vi "Post-Init.vi"(8 "error in (no error)":errorcluster, 11 "Pulse Driver in":refnum<class "Pulse Driver.lvclass">) -> (0 "error out":errorcluster, 2 "Init Result":refnum<class "Acquired Result.lvclass">, 3 "Pulse Driver out":refnum<class "Pulse Driver.lvclass">)   [LabVIEW 2019, in "Pulse Driver.lvclass"]
uses:
  Pulse Driver.lvclass
  Instrument Driver/Instrument Driver.lvclass
  Results/Acquired Result/Acquired Result.lvclass
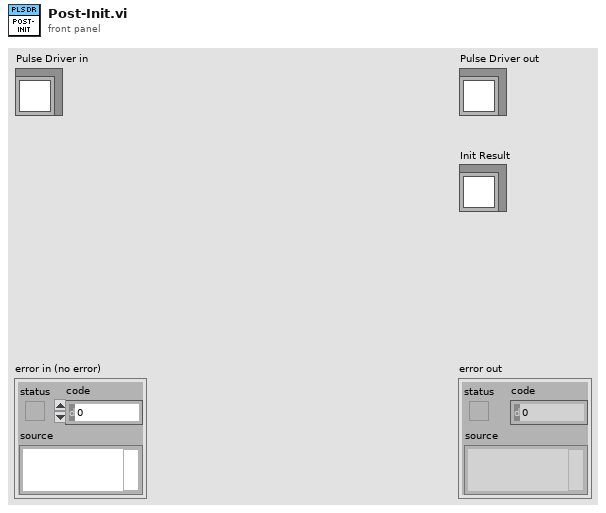
[diagram p1: front panel]
types:
  T1 = typedef "Pusle Driver Configuration.ctl" = cluster{"Pre-trigger duration":dbl, "Post-trigger duration":dbl, "Rate":dbl, "Ranges":dbl[], "Re-name channels":string[], "Active channels":string, "External clock":bool}
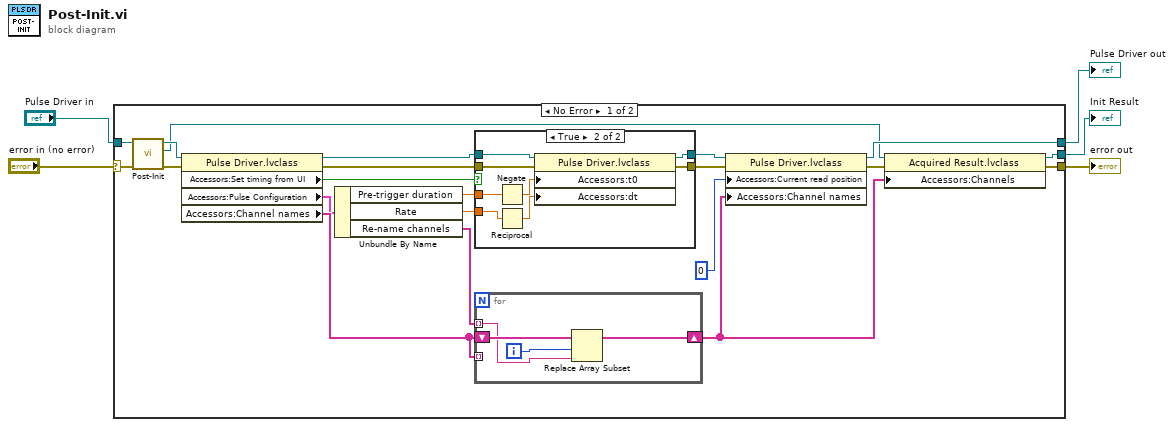
[diagram p0: block diagram]
diagram:
  n1 = case shown="No Error" "error in (no error)" {
    selector: "error in (no error)" -> [w16 w42]
    tunnel: [w21 w42] -> w4
    tunnel: [w26 w41] -> w2
    tunnel: "Pulse Driver in" -> [w24 w41]
    tunnel: [w19 _] -> w1
    frame No Error {
      n2 = call-parent "Post-Init.vi"("error in (no error)"=w16, "Instrument Driver in"=w24) -> ("error out"=w15:errorcluster, "Init Result"=w17:refnum<class "Acquired Result.lvclass">, "Instrument Driver out"=w18:refnum<class "Pulse Driver.lvclass">)  [unwired: 7 in]
      n3 = property class="Pulse Driver.lvclass"(reference=w18, error in=w15) -> (reference out=w13:refnum<class "Pulse Driver.lvclass">, error out=w10:errorcluster, "Accessors:Set timing from UI"=w6:bool, "Accessors:Pulse Configuration"=w7:T1, "Accessors:Channel names"=w8:string[])
      n4 = Unbundle By Name(w7) -> ("Pre-trigger duration"=w23:dbl, "Rate"=w22:dbl, "Re-name channels"=w9:string[])
      n5 = case shown="True" w6 {
        tunnel: w23 -> [_ w36]
        tunnel: w22 -> [_ w35]
        tunnel: w13 -> [w28 w32]
        tunnel: [w28 w31] -> w12
        tunnel: [w27 w30] -> w11
        tunnel: w10 -> [w27 w29]
        frame False {
        }
        frame True {
          n6 = Negate(x=w36) -> (-x=w34:dbl)
          n7 = Reciprocal(x=w35) -> (1/x=w33:dbl)
          n8 = property class="Pulse Driver.lvclass"(reference=w32, error in=w29, "Accessors:t0"=w34, "Accessors:dt"=w33) -> (reference out=w31:refnum<class "Pulse Driver.lvclass">, error out=w30:errorcluster)
        }
      }
      n9 = for {
        tunnel: w9 -> [w38] mode=indexing
        shift-right: [w37] -> w20
        shift-left: w8 -> [w40]
        tunnel: w8 -> [_] mode=indexing
        i -> [w39]
        n10 = Replace Array Subset(array=w40, new element=w38, index=w39) -> (w37:string[])
      }
      n11 = property class="Pulse Driver.lvclass"(reference=w12, error in=w11, "Accessors:Current read position"=0 ("Current read position"), "Accessors:Channel names"=w20) -> (reference out=w26:refnum<class "Pulse Driver.lvclass">, error out=w25:errorcluster)
      n12 = property class="Acquired Result.lvclass"(reference=w17, error in=w25, "Accessors:Channels"=w20) -> (reference out=w19:refnum<class "Acquired Result.lvclass">, error out=w21:errorcluster)
    }
    frame Error {
    }
  }
  "error out" <- w4
  "Pulse Driver out" <- w2
  "Init Result" <- w1
